vi "set_settings_cluster.vi"(8 "error in (no error)":errorcluster, 10 "settings cluster variant":variant, 11 "ImagingModeDL090130Frame in":refnum<class "ImagingModeDL090130Frame.lvclass">) -> (0 "error out":errorcluster, 3 "ImagingModeDL090130Frame out":refnum<class "ImagingModeDL090130Frame.lvclass">)   [LabVIEW 2010, in "ImagingModeDL090130Frame.lvclass"]
uses:
  ImagingModeDL090130Frame.lvclass
  ImagingModeDL090130Frame.lvclass/ImagingModeDL090130Frame.ctl
  common/xcontrols/XIntensityCompensation/XIntensityCompensation/XIntensityCompensation.xctl
  common/classes/ErrorController/ErrorController/class_data.vi
  common/classes/ErrorController/ErrorController/ErrorController.lvclass
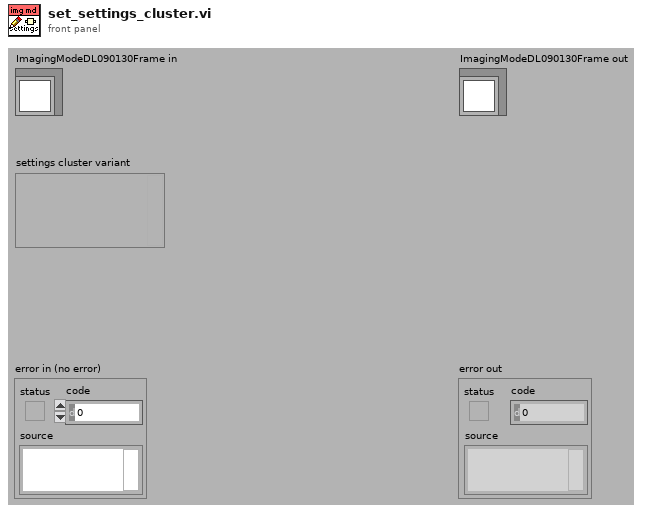
[diagram p1: front panel]
types:
  T1 = typedef "ImagingModeDL090130Frame.lvclass/settings_cluster.ctl" = cluster{"FrameSettings":cluster{"ResolutionX":i32, "ResolutionY":i32, "AspectRatioX":dbl, "AspectRatioY":dbl, "FrameScanRate":dbl[unit], "SpeedConstant":T2, "Vy0(V)":dbl, "deltaVy(V)":dbl, "Vz0(V)":dbl, "deltaVz(V)":dbl}, "StackSettings":cluster{"Frames":i32, "AveragingRepetitions":i32, "StepSize":dbl[unit], "ReturnToOrigin":bool, "TranslationMode":T3, "IntensityCompensationParameters":T4}}
  T2 = typedef "ImagingModeDL090130Frame.lvclass/speed_constant_enum.ctl" = enum16{"pixel dwell time", "line scan time", "frame rate"}
  T3 = typedef "ImagingModeDL090130Frame.lvclass/translation_mode_enum.ctl" = enum16{"scanHead", "stage"}
  T4 = typedef "XIntensityCompensation.xctl/data.ctl" = cluster{"A":dbl, "lambda":dbl[unit], "C":dbl}
  T5 = typedef "ImagingModeDL090130Frame.lvclass/control_refs.ctl" = cluster{"resolution controls":cluster{"x pixels":refnum<vi>, "y pixels":refnum<vi>, "ratio x factor":refnum<vi>, "ratio y factor":refnum<vi>, "center(xgalvo,V)":refnum<vi>, "center(ygalvo,V)":refnum<vi>, "amplitude(ygalvo,V)":refnum<vi>, "amplitude(xgalvo,V)":refnum<vi>}, "speed controls":cluster{"pixel dwell time":refnum<vi>, "line scan time":refnum<vi>, "frame rate":refnum<vi>, "keep constant":refnum<vi>}, "number of frames controls":cluster{"# of frames":refnum<vi>, "duration":refnum<vi>, "# of repetitions":refnum<vi>}, "current value indicators":cluster{"frame #":refnum<vi>, "repetition #":refnum<vi>, "offset":refnum<vi>}, "step controls":cluster{"step size":refnum<vi>, "return to origin?":refnum<vi>, "translation mode":refnum<vi>, "XIntensityCompensation":refnum<vi>}, "defineButton":refnum<vi>, "settings enforced?":refnum<vi>, "settings":refnum<vi>}
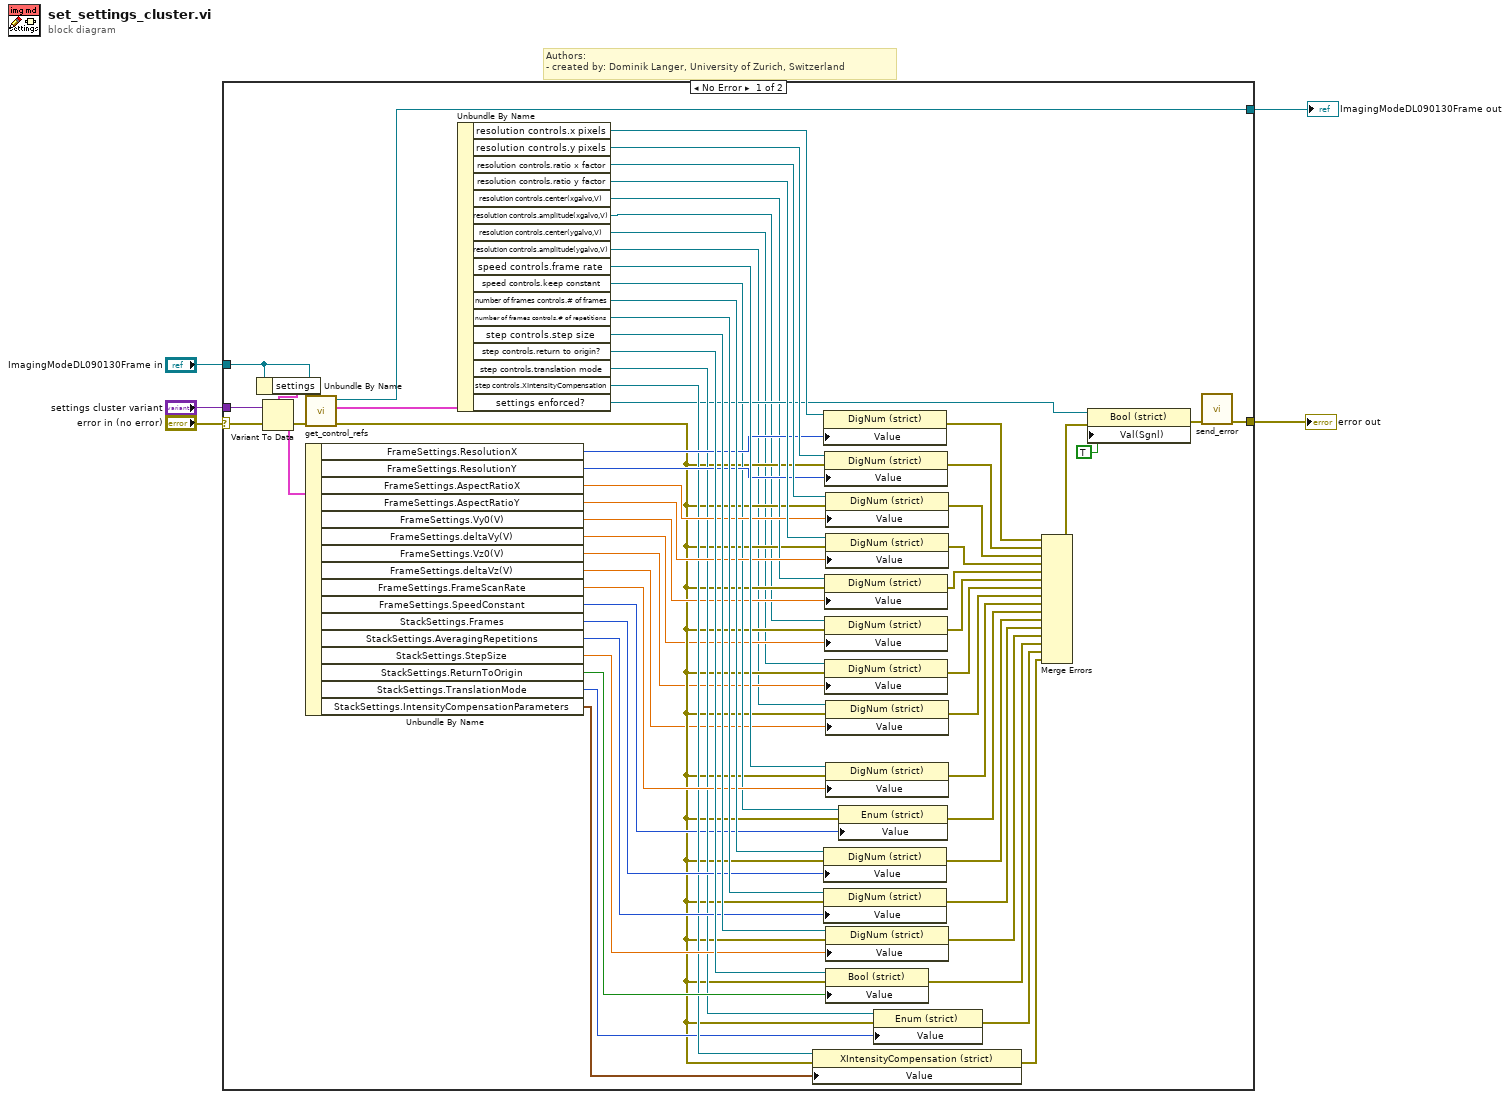
[diagram p0: block diagram]
diagram:
  # "Authors: \n- created by: Dominik Langer, University of Zurich, Switzerland"
  n1 = case shown="No Error" "error in (no error)" {
    selector: "error in (no error)" -> [w44 w69]
    tunnel: [w48 w69] -> w4
    tunnel: [w46 w68] -> w3
    tunnel: "ImagingModeDL090130Frame in" -> [w42 w68]
    tunnel: "settings cluster variant" -> [w43 _]
    frame No Error {
      n2 = Unbundle By Name(w42) -> ("settings"=w41:T1)
      n3 = Variant To Data(error in=w44, Variant=w43, type=w41) -> (error out=w47:errorcluster, data=w58:T1)
      n4 = call-dynamic "get_control_refs.vi"("error in (no error)"=w47, "ImagingModeDL090130Frame in"=w42) -> ("error out"=w20:errorcluster, "control refs"=w45:T5, "ImagingModeDL090130Frame out"=w46:refnum<class "ImagingModeDL090130Frame.lvclass">)  [unwired: 7 in]
      n5 = Unbundle By Name(w58) -> ("FrameSettings.ResolutionX"=w57:i32, "FrameSettings.ResolutionY"=w56:i32, "FrameSettings.AspectRatioX"=w55:dbl, "FrameSettings.AspectRatioY"=w54:dbl, "FrameSettings.Vy0(V)"=w21:dbl, "FrameSettings.deltaVy(V)"=w18:dbl, "FrameSettings.Vz0(V)"=w16:dbl, "FrameSettings.deltaVz(V)"=w14:dbl, "FrameSettings.FrameScanRate"=w53:dbl[unit], "FrameSettings.SpeedConstant"=w26:T2, "StackSettings.Frames"=w52:i32, "StackSettings.AveragingRepetitions"=w51:i32, "StackSettings.StepSize"=w50:dbl[unit], "StackSettings.ReturnToOrigin"=w49:bool, "StackSettings.TranslationMode"=w31:T3, "StackSettings.IntensityCompensationParameters"=w32:T4)
      n6 = Unbundle By Name(w45) -> ("resolution controls.x pixels"=w67:refnum<vi>, "resolution controls.y pixels"=w66:refnum<vi>, "resolution controls.ratio x factor"=w65:refnum<vi>, "resolution controls.ratio y factor"=w64:refnum<vi>, "resolution controls.center(xgalvo,V)"=w22:refnum<vi>, "resolution controls.amplitude(xgalvo,V)"=w19:refnum<vi>, "resolution controls.center(ygalvo,V)"=w17:refnum<vi>, "resolution controls.amplitude(ygalvo,V)"=w15:refnum<vi>, "speed controls.frame rate"=w63:refnum<vi>, "speed controls.keep constant"=w24:refnum<vi>, "number of frames controls.# of frames"=w62:refnum<vi>, "number of frames controls.# of repetitions"=w61:refnum<vi>, "step controls.step size"=w60:refnum<vi>, "step controls.return to origin?"=w59:refnum<vi>, "step controls.translation mode"=w35:refnum<vi>, "step controls.XIntensityCompensation"=w34:refnum<vi>, "settings enforced?"=w28:refnum<vi>)
      n7 = property class="XIntensityCompensation (strict)"(reference=w34, error in=w20, "Value"=w32) -> (error out=w33:errorcluster)  [unwired: 1 out]
      n8 = property class="DigNum (strict)"(reference=w67, "Value"=w57) -> (error out=w13:errorcluster)  [unwired: 1 in, 1 out]
      n9 = property class="DigNum (strict)"(reference=w62, error in=w20, "Value"=w52) -> (error out=w39:errorcluster)  [unwired: 1 out]
      n10 = property class="DigNum (strict)"(reference=w61, error in=w20, "Value"=w51) -> (error out=w38:errorcluster)  [unwired: 1 out]
      n11 = property class="DigNum (strict)"(reference=w66, error in=w20, "Value"=w56) -> (error out=w12:errorcluster)  [unwired: 1 out]
      n12 = property class="DigNum (strict)"(reference=w22, error in=w20, "Value"=w21) -> (error out=w6:errorcluster)  [unwired: 1 out]
      n13 = property class="DigNum (strict)"(reference=w19, error in=w20, "Value"=w18) -> (error out=w7:errorcluster)  [unwired: 1 out]
      n14 = property class="DigNum (strict)"(reference=w17, error in=w20, "Value"=w16) -> (error out=w8:errorcluster)  [unwired: 1 out]
      n15 = property class="DigNum (strict)"(reference=w65, error in=w20, "Value"=w55) -> (error out=w11:errorcluster)  [unwired: 1 out]
      n16 = property class="DigNum (strict)"(reference=w64, error in=w20, "Value"=w54) -> (error out=w10:errorcluster)  [unwired: 1 out]
      n17 = property class="DigNum (strict)"(reference=w15, error in=w20, "Value"=w14) -> (error out=w9:errorcluster)  [unwired: 1 out]
      n18 = property class="DigNum (strict)"(reference=w63, error in=w20, "Value"=w53) -> (error out=w40:errorcluster)  [unwired: 1 out]
      n19 = property class="DigNum (strict)"(reference=w60, error in=w20, "Value"=w50) -> (error out=w37:errorcluster)  [unwired: 1 out]
      n20 = property class="Bool (strict)"(reference=w59, error in=w20, "Value"=w49) -> (error out=w36:errorcluster)  [unwired: 1 out]
      n21 = property class="Enum (strict)"(reference=w24, error in=w20, "Value"=w26) -> (error out=w25:errorcluster)  [unwired: 1 out]
      n22 = property class="Enum (strict)"(reference=w35, error in=w20, "Value"=w31) -> (error out=w23:errorcluster)  [unwired: 1 out]
      n23 = Merge Errors(w13, w12, w11, w10, w6, w7, w8, w9, w40, w25, w39, w38, w37, w36, w23, w33) -> (w30:errorcluster)
      n24 = property class="Bool (strict)"(reference=w28, error in=w30, "Val(Sgnl)"=TRUE ("Value (Signaling)")) -> (error out=w29:errorcluster)  [unwired: 1 out]
      n25 = call "send_error.vi"("error in (no error)"=w29) -> ("error out"=w48:errorcluster)  [unwired: 10 in]
    }
    frame Error {
    }
  }
  "error out" <- w4
  "ImagingModeDL090130Frame out" <- w3
